vi "TestCloneRegClass.vi"() -> ()   [LabVIEW 2014, in "ModuleAdmin.lvlib"]
uses:
  ModuleAdmin.lvlib
  CloneRegistration.lvclass
panel:
  in  "IsFirst? Module ID":i32=101
  in  "Remove Module ID":i32=100
  in  "Second Module ID":i32=100
  in  "First Module ID":i32=101
  out "First?":bool=TRUE
  out "Found?":bool=TRUE
  out "ListFound":bool=TRUE
  out "Module IDs":i32[](array[numeric])=[101]
  out "First? (all)":bool[](array[boolean])=[TRUE]
  out "Instance Names":string[](array[string])=["101"]
  out "Removed":bool=TRUE
  out "error out":errorcluster
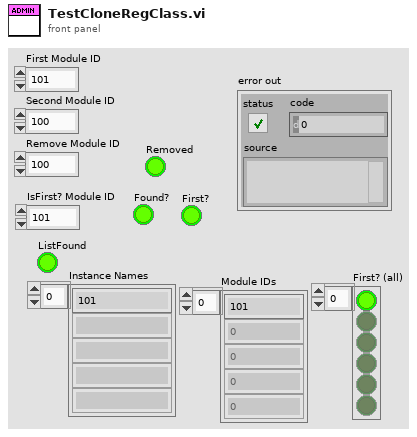
[diagram p1: front panel]
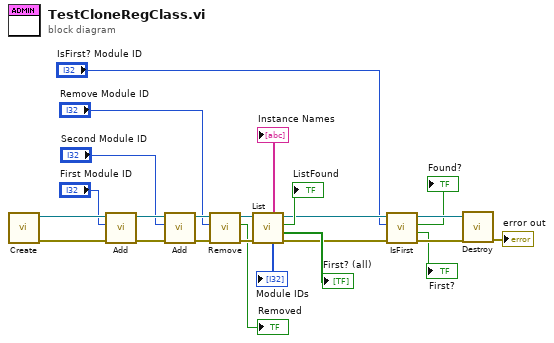
[diagram p0: block diagram]
diagram:
  n1 = call "Create.vi"() -> ("error out"=w22:errorcluster, "CloneRegRef"=w23:refnum<data-value>)  [unwired: 10 in]
  n2 = call "Add.vi"("error in (no error)"=w22, "Module ID"="First Module ID", "CloneRegRef"=w23) -> ("error out"=w17:errorcluster, "CloneRegRef"=w16:refnum<data-value>)  [unwired: 6 in, 1 out]
  n3 = call "Add.vi"("error in (no error)"=w17, "Module ID"="Second Module ID", "CloneRegRef"=w16) -> ("error out"=w14:errorcluster, "CloneRegRef"=w13:refnum<data-value>)  [unwired: 6 in, 1 out]
  n4 = call "Remove.vi"("error in (no error)"=w14, "Module ID"="Remove Module ID", "CloneRegRef"=w13) -> ("error out"=w12:errorcluster, "Found?"=→"Removed":bool, "CloneRegRef"=w11:refnum<data-value>)  [unwired: 6 in]
  n5 = call "List.vi"("error in (no error)"=w12, "CloneRegRef"=w11) -> ("error out"=w7:errorcluster, "First? (all)"=→"First? (all)":bool[], "Found?"=→"ListFound":bool, "CloneRegRef"=w6:refnum<data-value>, "Module IDs"=→"Module IDs":i32[], "Instance Names"=→"Instance Names":string[])  [unwired: 4 in]
  n6 = call "IsFirst.vi"("error in (no error)"=w7, "Module ID"="IsFirst? Module ID", "CloneRegRef"=w6) -> ("error out"=w5:errorcluster, "First?"=→"First?":bool, "Found?"=→"Found?":bool, "CloneRegRef"=w4:refnum<data-value>)  [unwired: 5 in]
  n7 = call "Destroy.vi"("error in (no error)"=w5, "CloneRegRef"=w4) -> ("error out"=→"error out":errorcluster)  [unwired: 9 in]
